vi "ParseHierarchyProps.vi"(10 "Number of Channels":i32, 11 "Lines":T1[](array[typedef])) -> (3 "Array of Hierarchy Properties":string[][](array[string]))   [LabVIEW 2017]
uses:
  <vilib>/addons/InsightCM/Utilities/TDMSFileGenerator/controls/Hierarchy_Line.ctl
  <vilib>/addons/InsightCM/Utilities/TDMSFileGenerator/controls/Hierarchy_Equipment.ctl
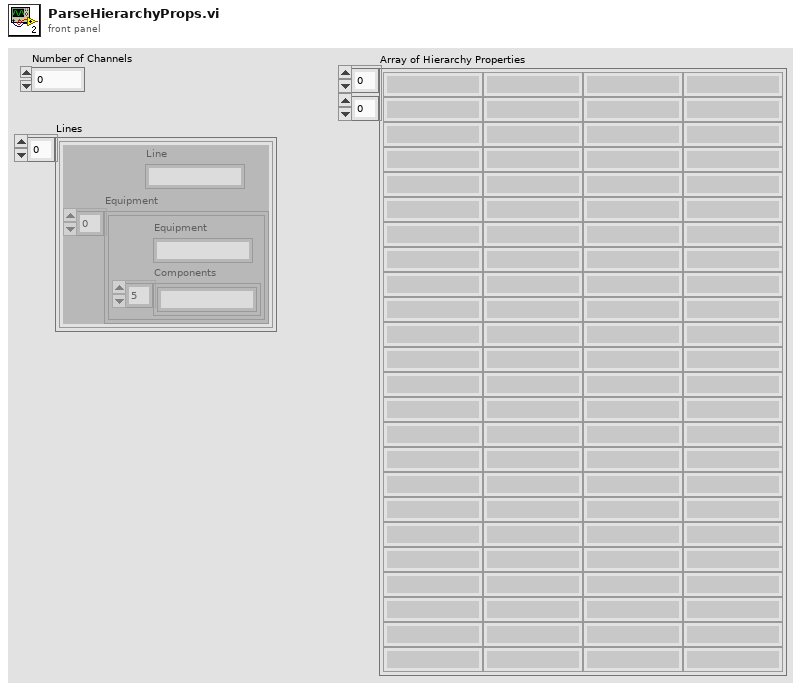
[diagram p1: front panel]
types:
  T1 = typedef "Hierarchy_Line.ctl" = cluster{"Line":string, "Equipment":T2[]}
  T2 = typedef "Hierarchy_Equipment.ctl" = cluster{"Equipment":string, "Components":string[]}
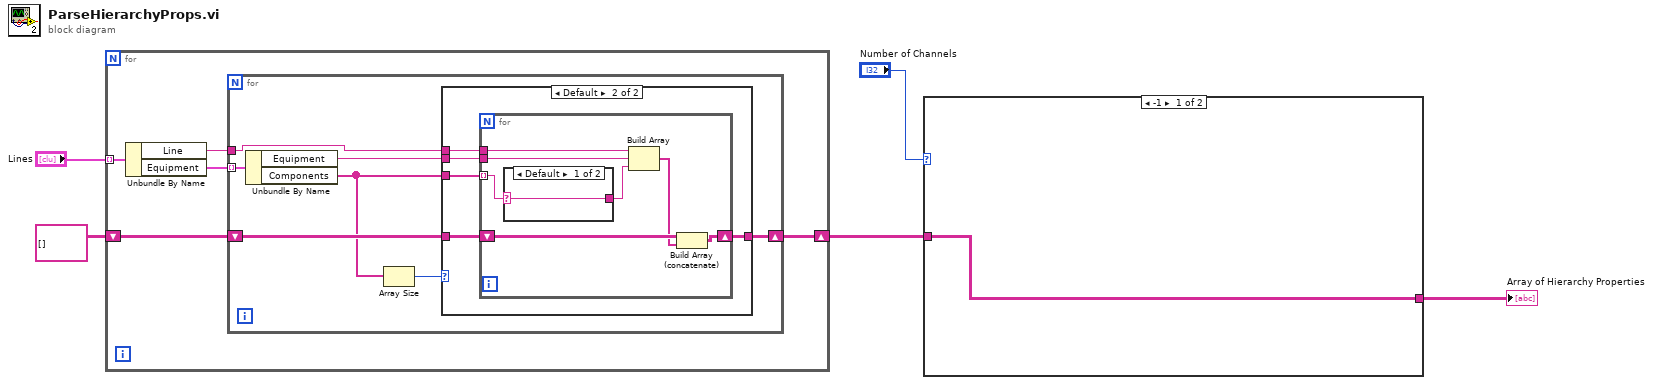
[diagram p0: block diagram]
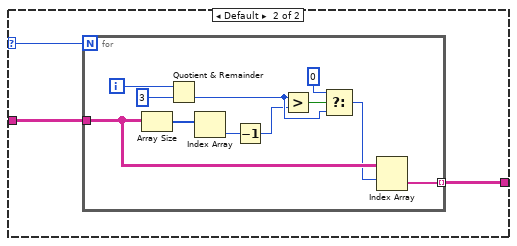
[diagram p2: hidden frame]
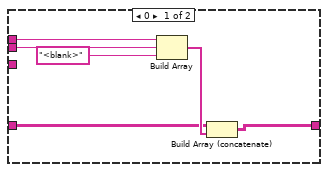
[diagram p3: hidden frame]
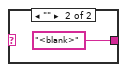
[diagram p4: hidden frame]
diagram:
  n1 = for {
    tunnel: "Lines" -> [w10] mode=indexing
    shift-right: [w6] -> w3
    shift-left: string[][] [] -> [w7]
    n2 = Unbundle By Name(w10) -> ("Line"=w9:string, "Equipment"=w8:T2[])
    n3 = for {
      tunnel: w9 -> [w16]
      tunnel: w8 -> [w17] mode=indexing
      shift-right: [w13] -> w6
      shift-left: w7 -> [w14]
      n4 = Unbundle By Name(w17) -> ("Equipment"=w15:string, "Components"=w12:string[])
      n5 = Array Size(array=w12) -> (size(s)=w11:i32)
      n6 = case shown="Default" w11 {
        tunnel: w12 -> [_ w28]
        tunnel: w16 -> [w22 w27]
        tunnel: w15 -> [w21 w26]
        tunnel: w14 -> [w19 w25]
        tunnel: [w20 w24] -> w13
        frame 0 {
          n7 = Build Array(w22, w21, "<blank>" ("element")) -> (w23:string[])
          n8 = Build Array (concatenate)(w19, w23) -> (w20:string[][])
        }
        frame Default {
          n9 = for {
            tunnel: w28 -> [w30] mode=indexing
            tunnel: w27 -> [w35]
            tunnel: w26 -> [w34]
            shift-right: [w31] -> w24
            shift-left: w25 -> [w33]
            n10 = case shown="Default" w30 {
              selector: w30 -> [w36 _]
              tunnel: [w36 "<blank>" ("element")] -> w29
              frame Default {
              }
              frame "" {
              }
            }
            n11 = Build Array(w35, w34, w29) -> (w32:string[])
            n12 = Build Array (concatenate)(w33, w32) -> (w31:string[][])
          }
        }
      }
    }
  }
  n13 = case shown="-1" "Number of Channels" {
    selector: "Number of Channels" -> [_ w39]
    tunnel: w3 -> [w38 w41]
    tunnel: [w38 w40] -> w2
    frame -1 {
    }
    frame Default {
      n14 = for {
        N: w39 -> [_]
        tunnel: w41 -> [w44]
        tunnel: [w42] -> w40 mode=indexing
        i -> [w45]
        n15 = Array Size(array=w44) -> (size(s)=w51:i32[])
        n16 = Quotient & Remainder(x=w45, y=3) -> (floor(x/y)=w48:i32)  [unwired: 1 out]
        n17 = Index Array(array=w51) -> (element=w47:i32)  [unwired: 1 in]
        n18 = Decrement(x=w47) -> (x-1=w46:i32)
        n19 = Greater?(x=w48, y=w46) -> (0:w50:bool)
        n20 = Select(t=0, s=w50, f=w48) -> (s? t:f=w43:i32)
        n21 = Index Array(array=w44, index (row)=w43) -> (element=w42:string[])  [unwired: 1 in]
      }
    }
  }
  "Array of Hierarchy Properties" <- w2
